vi "Initialize Serial.vi"(8 "error in (no error)":errorcluster, 11 "VISA resource name":refnum<visa-resource-name>) -> (0 "error out":errorcluster, 3 "VISA resource name out":refnum<visa-resource-name>)   [LabVIEW 2019, in "PGC2D.lvlib"]
uses:
  PGC2D.lvlib
  Program Files (x86)/National Instruments/LabVIEW 2019/examples/Instrument IO/Serial/support/Serial - Settings.ctl
  <vilib>/Instr/_visa.llb/VISA Configure Serial Port (Instr).vi
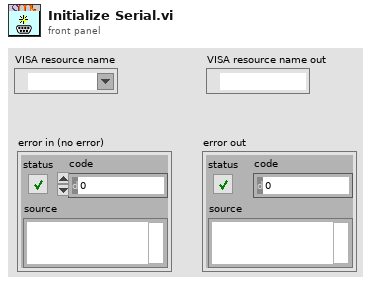
[diagram p1: front panel]
types:
  T1 = typedef "Serial - Settings.ctl" = cluster{"baud rate":u32, "data bits":u16, "parity":enum16{"None", "Odd", "Even", "Mark", "Space"}, "stop bits":u16, "flow control":u16}
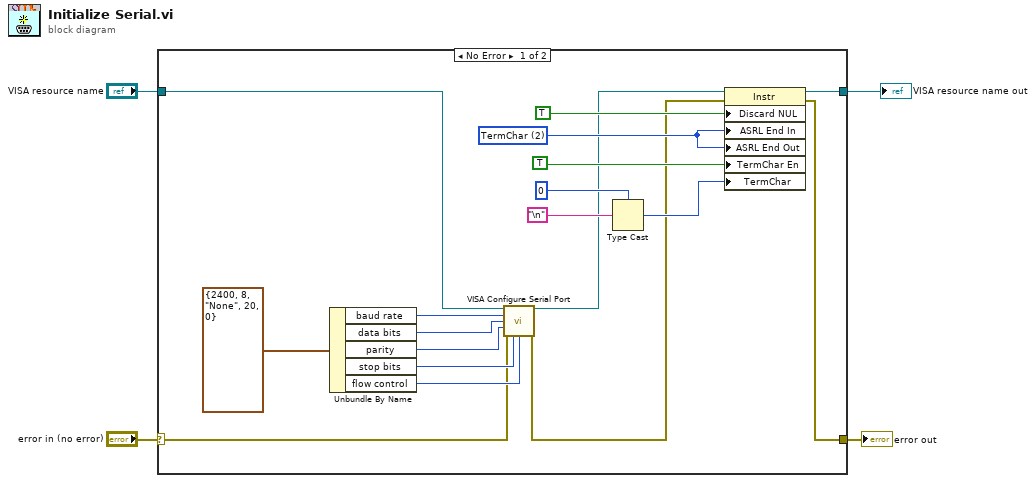
[diagram p0: block diagram]
diagram:
  n1 = case shown="No Error" "error in (no error)" {
    selector: "error in (no error)" -> [w10 w23]
    tunnel: "VISA resource name" -> [w5 w24]
    tunnel: [w6 w23] -> w3
    tunnel: [w7 w24] -> w2
    frame No Error {
      w17 = u16 2 items=["None", "Last Bit", "TermChar"] ("Serial Settings:End Mode for Reads")
      n2 = Unbundle By Name(T1 {"baud rate"=2400, "data bits"=8, "parity"=enum."None", "stop bits"=20, "flow control"=0} ("input cluster")) -> ("baud rate"=w12:u32, "data bits"=w13:u16, "parity"=w14:enum16{"None", "Odd", "Even", "Mark", "Space"}, "stop bits"=w15:u16, "flow control"=w16:u16)
      n3 = call-poly "VISA Configure Serial Port"("VISA resource name"=w5, "baud rate (9600)"=w12, "data bits (8)"=w13, "parity (0:none)"=w14, "error in (no error)"=w10, "stop bits (10: 1 bit)"=w15, "flow control (0:none)"=w16) -> ("VISA resource name out"=w9:refnum<visa-resource-name>, "error out"=w8:errorcluster)  [unwired: 7 in]
      n4 = Type Cast(type=u8 0, x="\n") -> (*(type *) &x=w20:u8)
      n5 = property class="Instr"(reference=w9, error in=w8, "Discard NUL"=TRUE ("Serial Settings:Discard NUL Characters"), "ASRL End In"=w17, "ASRL End Out"=w17, "TermChar En"=TRUE ("Message Based Settings:Termination Character Enable"), "TermChar"=w20) -> (reference out=w7:refnum<visa-resource-name>, error out=w6:errorcluster)
    }
    frame Error {
    }
  }
  "error out" <- w3
  "VISA resource name out" <- w2
